vi "Configure Port by Index.vi"(6 "msg count":u32, 8 "error in (no error)":errorcluster, 9 "handle":u32, 10 "Index":i32, 11 "ubrx in":T1) -> (0 "error out":errorcluster, 3 "ubrx out":T1)   [LabVIEW 2020, in "UdpBlockMessage.lvlib"]
uses:
  UdpBlockMessage.lvlib
  _typdefes/UdpBlockReadInPort_type.ctl
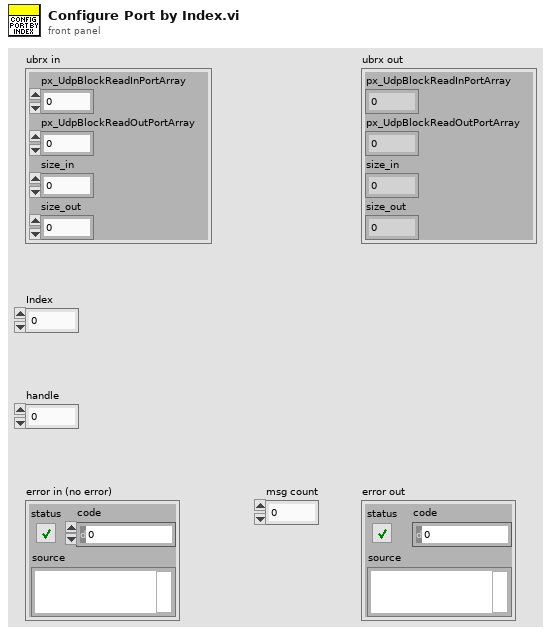
[diagram p1: front panel]
types:
  T1 = cluster{"px_UdpBlockReadInPortArray":u64, "px_UdpBlockReadOutPortArray":u64, "size_in":i32, "size_out":i32}
  T2 = typedef "UdpBlockMessage.lvlib/UdpBlockReadInPort_type.ctl" = cluster{"ul_UdpHandle":u32, "ul_MsgCount":u32}
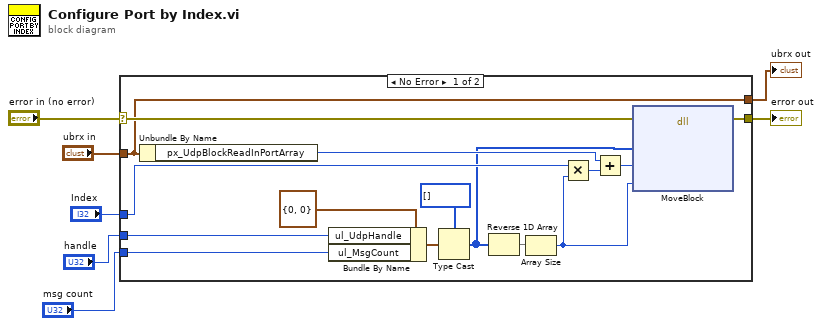
[diagram p0: block diagram]
diagram:
  n1 = case shown="No Error" "error in (no error)" {
    selector: "error in (no error)" -> [w15 w24]
    tunnel: [w14 w24] -> w6
    tunnel: "Index" -> [w17 _]
    tunnel: "ubrx in" -> [w11 w23]
    tunnel: "handle" -> [w21 _]
    tunnel: "msg count" -> [w20 _]
    tunnel: [w11 w23] -> w1
    frame No Error {
      n2 = Unbundle By Name(w11) -> ("px_UdpBlockReadInPortArray"=w10:u64)
      n3 = Bundle By Name(cluster=T2 {"ul_UdpHandle"=0, "ul_MsgCount"=0} ("UdpBlockReadInPort"), "ul_UdpHandle"=w21, "ul_MsgCount"=w20) -> (w19:T2)
      n4 = Type Cast(type=u8[] [], x=w19) -> (*(type *) &x=w9:u8[])
      n5 = Reverse 1D Array(array=w9) -> (reversed array=w8:u8[])
      n6 = Array Size(array=w8) -> (size(s)=w16:i32)
      n7 = Multiply(x=w17, y=w16) -> (x*y=w13:i32)
      n8 = Add(x=w10, y=w13) -> (x+y=w12:u64)
      n9 = dll-call lib="LabVIEW" fn="MoveBlock"(error in=w15, "src"=w9, "dst"=w12, "size"=w16) -> (error out=w14:errorcluster)  [unwired: 6 in, 1 out]
    }
    frame Error {
    }
  }
  "error out" <- w6
  "ubrx out" <- w1
